vi "SSL_set_tlsext_host_name.vi"(8 "error in (no error)":errorcluster, 10 "Hostname":string="localhost", 11 "SSL in":refnum<class "SSL.lvclass">) -> (0 "error out":errorcluster, 3 "SSL out":refnum<class "SSL.lvclass">)   [LabVIEW 2013, in "SSL_Lib.lvlib" / "SSL.lvclass"]
uses:
  SSL.lvclass
  SSL-Lib/SSL-Lib.lvclass/SSL-Lib.ctl
  SSL.lvclass/SSL.ctl
  SSL-Lib/Read SSL Library Path.vi
  Read Handle.vi
  SSL-Lib/SSL-Lib.lvclass
panel:
  out "return type":i32
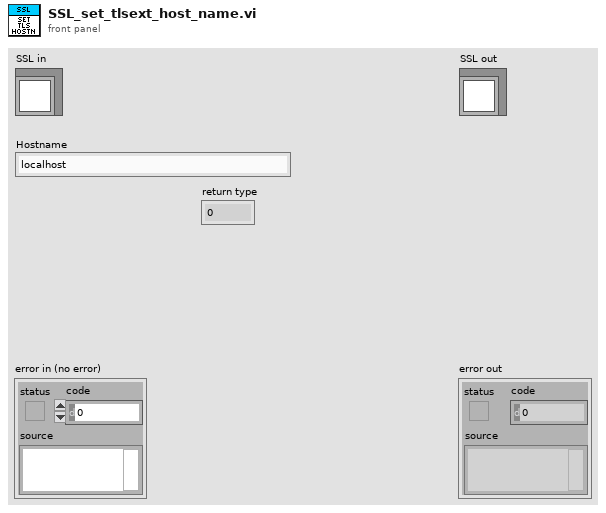
[diagram p1: front panel]
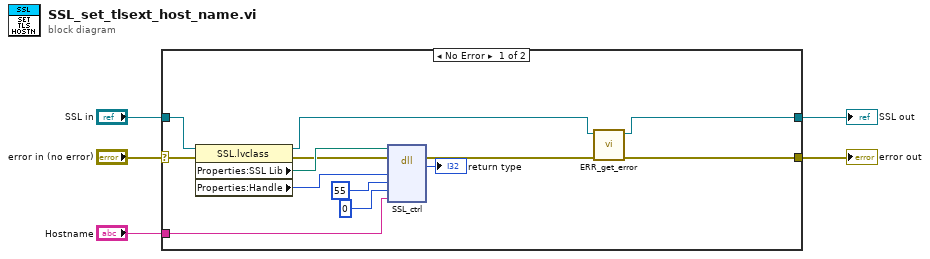
[diagram p0: block diagram]
diagram:
  n1 = case shown="No Error" "error in (no error)" {
    selector: "error in (no error)" -> [w17 w20]
    tunnel: [w8 w20] -> w4
    tunnel: [w6 w19] -> w2
    tunnel: "SSL in" -> [w18 w19]
    tunnel: "Hostname" -> [w13 _]
    frame No Error {
      n2 = property class="SSL.lvclass"(reference=w18, error in=w17) -> (reference out=w7:refnum<class "SSL.lvclass">, error out=w15:errorcluster, "Properties:SSL Lib"=w16:path, "Properties:Handle"=w12:u64)
      n3 = dll-call lib="C:/Program Files (x86)/National Instruments/Shared/nissl/NIssleay32.dll" fn="SSL_ctrl"(path in=w16, error in=w15, "SSL"=w12, "cmd"=55, "larg"=0, "parg"=w13) -> (error out=w14:errorcluster, "return type"=→"return type":i32)  [unwired: 5 in, 1 out]
      n4 = call "ERR_get_error.vi"("error in (no error)"=w14, "SSL-Lib in"=w7) -> ("error out"=w8:errorcluster, "SSL-Lib out"=w6:refnum<class "SSL.lvclass">)  [unwired: 8 in]
    }
    frame Error {
    }
  }
  "error out" <- w4
  "SSL out" <- w2
